vi "03-without_args_and_returned_val.vi"() -> ()   [LabVIEW 2018, in "LV-0mq-Julia_roundtrip-lib.lvlib"]
uses:
  LV-0mq-Julia_roundtrip-lib.lvlib
  Server or client state.ctl
  detailed error info.ctl
  StackFrame.ctl
  Commands.ctl
  3a82b6dd-e193-42c5-8b03-f24c274193dd.vi
  3a82b6dd-e193-42c5-8b03-f24c274193dd.vi/ee143c56-f157-43d0-9360-6e82c2bc6abe.vi
  3a82b6dd-e193-42c5-8b03-f24c274193dd.vi/ee143c56-f157-43d0-9360-6e82c2bc6abe.vi/04d628df-8c73-4936-a8c8-ec903ac7e8dc.vi
  3a82b6dd-e193-42c5-8b03-f24c274193dd.vi/ee143c56-f157-43d0-9360-6e82c2bc6abe.vi/456f91f7-bce2-4f08-9ef6-35fb245e7a0b.vi
  3a82b6dd-e193-42c5-8b03-f24c274193dd.vi/ee143c56-f157-43d0-9360-6e82c2bc6abe.vi/737b7918-d5e8-4dee-b212-30beb2f2f348.vi
  jl-scripts path.vi
  check ID validity.vi
  bindata_descr to JSON.vi
  check cluster field names.vi
  concat JSON.vi
  build request.vi
  Parse server response.vi
  log jl exceptions.vi
panel:
  in  "next":bool
  out "detailed error info":T1
  out "current error":errorcluster
  out "final error":errorcluster
  out "short err code":u8
  in  "stop":bool
  out "ZMQ timeout":bool
  out "Julia script file path":path
  out "temporary script path":path
  out "Jl Server state":T3
  # "No arguments are sent and no values recieved here. The Julia script should each time print \"Hello World!\" in the terminal window."
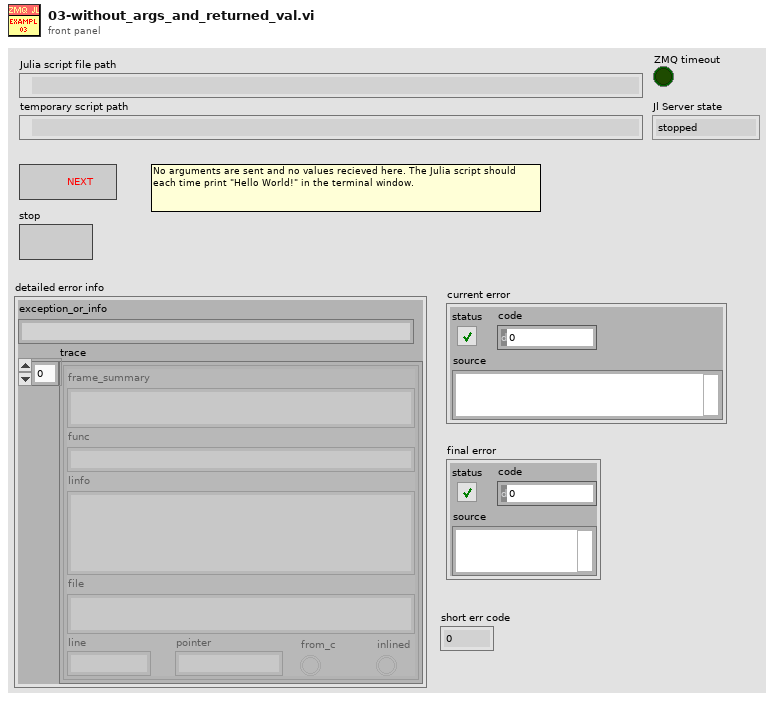
[diagram p1: front panel]
types:
  T1 = typedef "LV-0mq-Julia_roundtrip-lib.lvlib/detailed error info.ctl" = cluster{"exception_or_info":string, "trace":T2[]}
  T2 = typedef "LV-0mq-Julia_roundtrip-lib.lvlib/StackFrame.ctl" = cluster{"frame_summary":string, "func":string, "linfo":string, "file":string, "line":i32, "pointer":u64, "from_c":bool, "inlined":bool}
  T3 = typedef "LV-0mq-Julia_roundtrip-lib.lvlib/Server or client state.ctl" = enum16{"stopped", "running", "unknown"}
  T4 = typedef "LV-0mq-Julia_roundtrip-lib.lvlib/Commands.ctl" = enum16{"Start Jl-server & Init LV-client", "Send request & Get response ", "Stop Jl-server & Cleanup LV-client", "Cleanup LV-client", "Start Jl-server", "Stop Jl-server", "Init LV-Client", "Cleanup LV-Client", "(not allowed)", "Set LV Client state", "Set Jl Server state", "set ZMQ timeout", "read ZMQ timeout", "read-out state"}
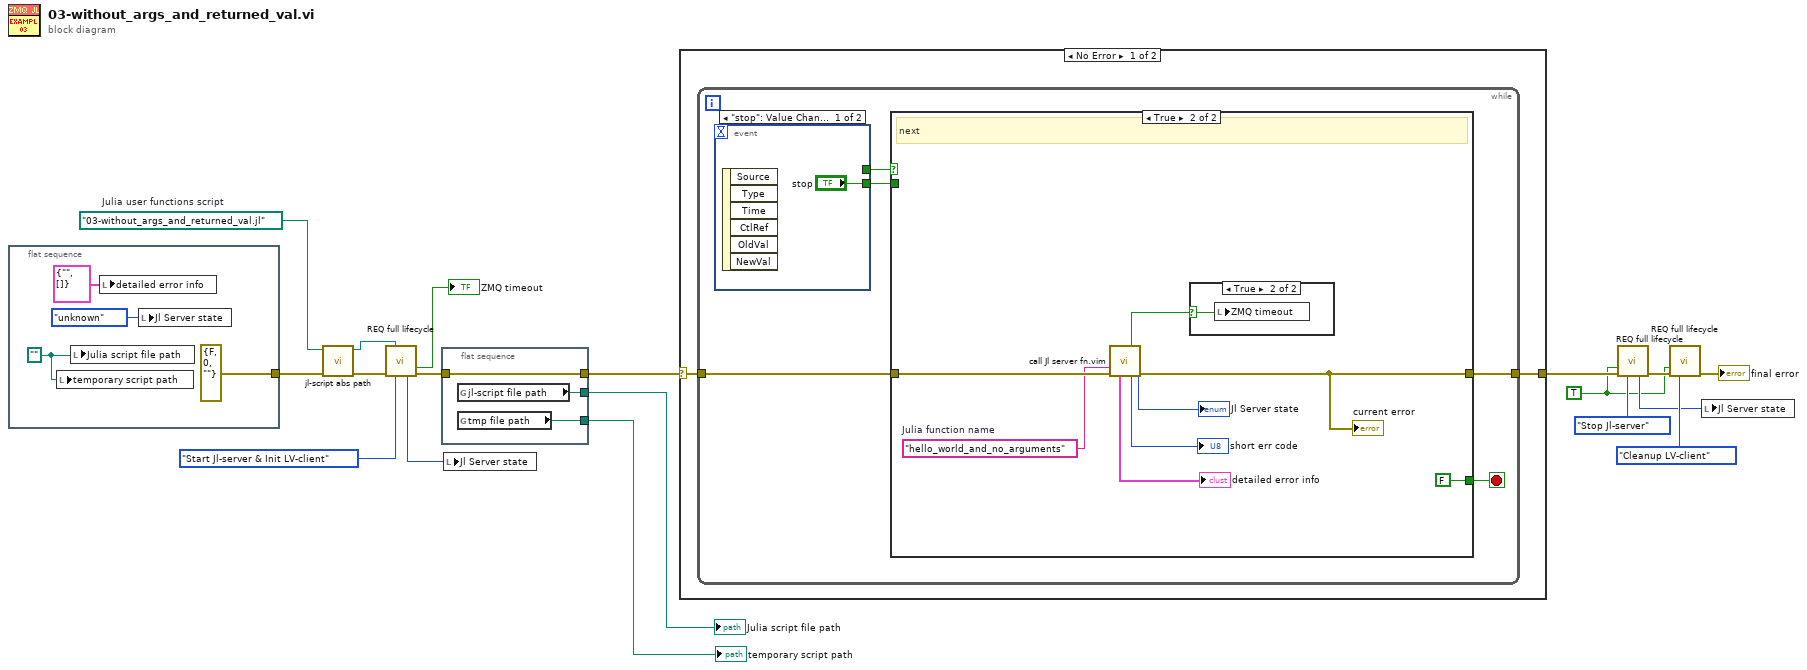
[diagram p0: block diagram]
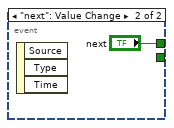
[diagram p2: hidden frame]
diagram:
  w4 = path "03-without_args_and_returned_val.jl"  # Julia user functions script
  w1 = TRUE ("Force command")
  n1 = flat-sequence {
    tunnel: [errorcluster {"status"=FALSE, "code"=0, "source"=""} ("error in (no error)")] -> w2
    frame #0 {
      w19 = path ""
      n2 = local write "temporary script path"(w19) -> ()
      n3 = local write "Julia script file path"(w19) -> ()
      n4 = local write "detailed error info"(T1 {"exception_or_info"="", "trace"=[]} ("detailed error info")) -> ()
      n5 = local write "Jl Server state"(Server_or_client_state."unknown" ("Jl Server state out")) -> ()
    }
  }
  n6 = call "jl-script abs path.vi"("error in (no error)"=w2, "Julia user functions script"=w4) -> ("error out"=w5:errorcluster, "script abs path"=w6:path)  [unwired: 8 in]
  n7 = call "REQ full lifecycle.vi"("Julia user functions script"=w6, "error in"=w5, "command"=Commands."Start Jl-server & Init LV-client") -> ("timeout?"=→"ZMQ timeout":bool, "Jl Server state out"=w8:T3, "error out"=w7:errorcluster)  [unwired: 6 in, 4 out]
  n8 = flat-sequence {
    tunnel: [w25] -> w13
    tunnel: w7 -> [w25]
    tunnel: [w24] -> w11
    tunnel: [w23] -> w12
    frame #0 {
      n9 = global read "jl-scripts path.vi" "jl-script file path"() -> (w24:path)
      n10 = global read "jl-scripts path.vi" "tmp file path"() -> (w23:path)
    }
  }
  n11 = local write "Jl Server state"(w8) -> ()
  n12 = case shown="No Error" w13 {
    selector: w13 -> [w26 w46]
    tunnel: [w27 w46] -> w18
    frame No Error {
      n13 = while {
        tunnel: w26 -> [w31]
        tunnel: [w32] -> w27
        stop <- w29 stop-if-true
        n14 = event shown="[0] \"stop\": Value Change" {
          selector: _ -> [_ _]
          dyn-events: _ -> [_ _]
          timeout: _ -> [_ _]
          tunnel: [_ "next"] -> w30
          tunnel: ["stop" _] -> w28
          event "stop": Value Change {
            n15 = event-data() -> ()  [unwired: 1 in, 6 out]
          }
          event "next": Value Change {
            n16 = event-data() -> ()  [unwired: 1 in, 3 out]
          }
        }
        n17 = case shown="True" w30 {
          tunnel: [w36 w42] -> w32
          tunnel: w31 -> [w36 w43]
          tunnel: [w35 FALSE ("stop this VI only")] -> w29
          tunnel: w28 -> [w35 _]
          frame False {
            # "stop"
          }
          frame True {
            w40 = "hello_world_and_no_arguments"  # Julia function name
            # "next"
            n18 = call "call Jl server fn.vim"("fun2call"=w40, "error in (no error)"=w43) -> ("timeout?"=w41:bool, "Jl Server state out"=→"Jl Server state":T3, "detailed error info"=→"detailed error info":T1, "return code"=→"short err code":u8, "error out"=w42:errorcluster)  [unwired: 7 in, 2 out]
            "current error" <- w42
            n19 = case shown="True" w41 {
              selector: w41 -> [_ w45]
              frame False {
              }
              frame True {
                n20 = local write "ZMQ timeout"(w45) -> ()
              }
            }
          }
        }
      }
    }
    frame Error {
    }
  }
  n21 = call "REQ full lifecycle.vi"("Force command"=w1, "error in"=w18, "command"=Commands."Stop Jl-server") -> ("Jl Server state out"=w10:T3, "error out"=w16:errorcluster)  [unwired: 6 in, 5 out]
  n22 = call "REQ full lifecycle.vi"("Force command"=w1, "error in"=w16, "command"=Commands."Cleanup LV-client") -> ("error out"=→"final error":errorcluster)  [unwired: 6 in, 6 out]
  n23 = local write "Jl Server state"(w10) -> ()
  "temporary script path" <- w12
  "Julia script file path" <- w11
